vi "manage data files.vi"(8 "error in":errorcluster, 9 "tracking":bool, 10 "recording type":enum16{"tracking", "stage"}(ring), 11 "refnum in":refnum<file>) -> (0 "error out":errorcluster, 1 "file open for writing":bool, 2 "file access error":bool, 3 "refnum out":refnum<file>)   [LabVIEW 2010]
uses:
  tracking and stage files global.vi
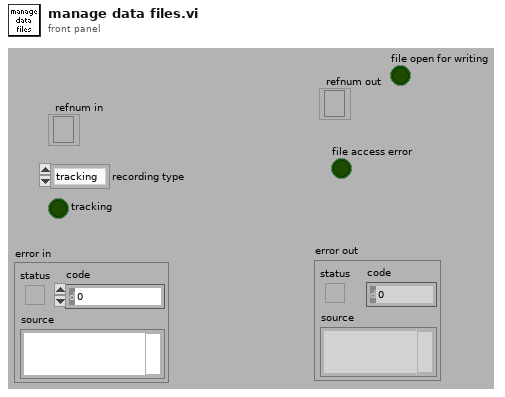
[diagram p1: front panel]
types:
  T1 = enum16{"open", "replace", "create", "open or create", "replace or create", "replace or create with confirmation"}
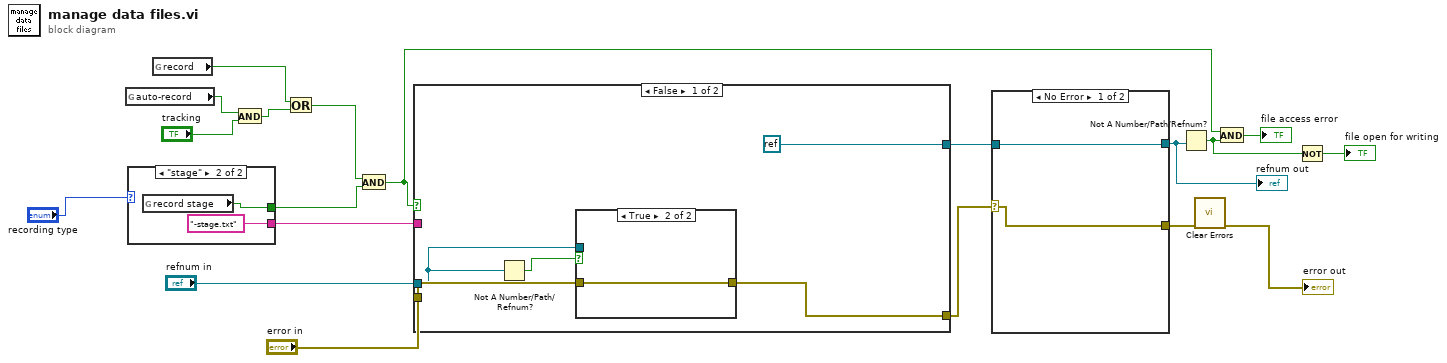
[diagram p0: block diagram]
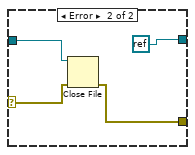
[diagram p2: hidden frame]
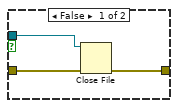
[diagram p3: hidden frame]
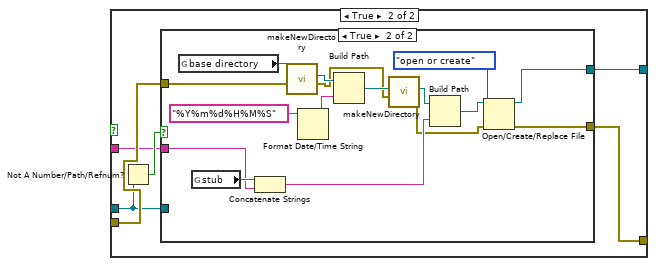
[diagram p4: hidden frame]
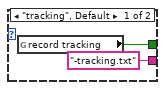
[diagram p6: hidden frame]
diagram:
  n1 = global read "tracking and stage files global.vi" "auto-record"() -> (w19:bool)
  n2 = case shown="\"stage\"" "recording type" {
    tunnel: [w21 w23] -> w13
    tunnel: ["-tracking.txt" "-stage.txt"] -> w11
    frame "tracking", Default {
      n3 = global read "tracking and stage files global.vi" "record tracking"() -> (w21:bool)
    }
    frame "stage" {
      n4 = global read "tracking and stage files global.vi" "record stage"() -> (w23:bool)
    }
  }
  n5 = global read "tracking and stage files global.vi" "record"() -> (w16:bool)
  n6 = And(x=w19, y="tracking") -> (x .and. y?=w17:bool)
  n7 = Or(x=w16, y=w17) -> (x .or. y?=w14:bool)
  n8 = And(x=w14, y=w13) -> (x .and. y?=w5:bool)
  n9 = case shown="False" w5 {
    tunnel: "refnum in" -> [w26 w33]
    tunnel: w11 -> [_ w36]
    tunnel: "error in" -> [w28 w37]
    tunnel: [w25 w34] -> w9
    tunnel: [refnum<k0> refnum w35] -> w8
    frame False {
      n10 = Not A Number/Path/Refnum?(number/path/refnum=w26) -> (NaN/Path/Refnum?=w27:bool)
      n11 = case shown="True" w27 {
        tunnel: w28 -> [w31 w32]
        tunnel: w26 -> [w30 _]
        tunnel: [w29 w32] -> w25
        frame False {
          n12 = Close File(refnum=w30, error in=w31) -> (error out=w29:errorcluster)  [unwired: 1 out]
        }
        frame True {
        }
      }
    }
    frame True {
      n13 = Not A Number/Path/Refnum?(number/path/refnum=w33) -> (NaN/Path/Refnum?=w38:bool)
      n14 = case shown="True" w38 {
        tunnel: w37 -> [w40 w50]
        tunnel: w36 -> [_ w47]
        tunnel: [w39 w42] -> w35
        tunnel: [w40 w41] -> w34
        tunnel: w33 -> [w39 _]
        frame False {
        }
        frame True {
          n15 = global read "tracking and stage files global.vi" "base directory"() -> (w56:path)
          n16 = global read "tracking and stage files global.vi" "stub"() -> (w49:string)
          n17 = Concatenate Strings(w49, w47) -> (w46:string)
          n18 = call "makeNewDirectory.vi"("error in (no error)"=w50, "path"=w56) -> ("error out"=w51:errorcluster, "path out"=w55:path)  [unwired: 8 in]
          n19 = Format Date/Time String(time format string (%c)="%Y%m%d%H%M%S") -> (date/time string=w53:string)  [unwired: 2 in]
          n20 = Build Path(base path=w55, name or relative path=w53) -> (appended path=w52:path)
          n21 = call "makeNewDirectory.vi"("error in (no error)"=w51, "path"=w52) -> ("error out"=w43:errorcluster, "path out"=w48:path)  [unwired: 8 in]
          n22 = Build Path(base path=w48, name or relative path=w46) -> (appended path=w45:path)
          n23 = Open/Create/Replace File(file path (use dialog)=w45, error in=w43, operation (0:open)=T1."open or create") -> (refnum out=w42:refnum<file>, error out=w41:errorcluster)  [unwired: 3 in, 1 out]
        }
      }
    }
  }
  n24 = case shown="No Error" w9 {
    selector: w9 -> [w57 w62]
    tunnel: [w58 refnum<k0> refnum] -> w6
    tunnel: w8 -> [w58 w59]
    tunnel: [w57 w61] -> w7
    frame No Error {
    }
    frame Error {
      n25 = Close File(refnum=w59, error in=w62) -> (error out=w61:errorcluster)  [unwired: 1 out]
    }
  }
  "refnum out" <- w6
  n26 = Not A Number/Path/Refnum?(number/path/refnum=w6) -> (NaN/Path/Refnum?=w2:bool)
  n27 = call <vilib>:"Clear Errors.vi"("error in (no error)"=w7) -> ("error out"=→"error out":errorcluster)  [unwired: 6 in]
  n28 = And(x=w5, y=w2) -> (x .and. y?=→"file access error":bool)
  n29 = Not(x=w2) -> (.not. x?=→"file open for writing":bool)
